vi "Equal To Core Actor.vi"(7 "Actor":refnum<class "Actor.lvclass">) -> (2 "Core Actor":bool)   [LabVIEW 2025, in "jettl.lvlib"]
uses:
  jettl.lvlib
  Actor/Actor/Actor.lvclass
  Actor/Actor.lvlib
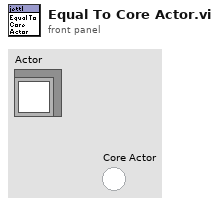
[diagram p1: front panel]
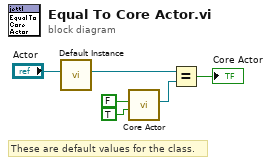
[diagram p0: block diagram]
diagram:
  # "These are default values for the class."
  n1 = call "Default Instance.vi"("Instance"="Actor") -> ("Default Instance"=w1:refnum<class "Actor.lvclass">)  [unwired: 10 in]
  n2 = call "Core Actor.vi"("Stop When Parent Stopped"=TRUE, "Root"=FALSE) -> ("Actor"=w5:refnum<class "Actor.lvclass">)  [unwired: 9 in]
  n3 = Equal?(x=w1, y=w5) -> (x = y?=→"Core Actor":bool)
